vi "AAL NB Filter Specification.vi"(8 "timing jitter":enum32{"Interpolation", "Rounding"}(ring), 9 "stop band attenuation":dbl=2.0 format="%.2f", 11 "maximum decimation factor":i32) -> (1 "A stop [dB]":dbl=72.0 format="%.2f", 3 "decimation factor":i32)   [LabVIEW 2014, in "NI_AALPro.lvlib"]
uses:
  NI_AALPro.lvlib
panel:
  in  "force power of 2?":bool
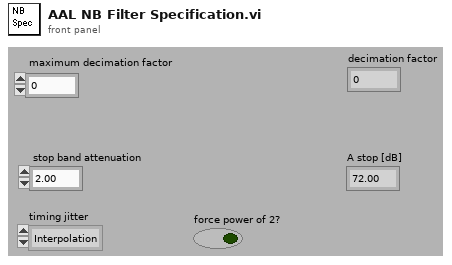
[diagram p1: front panel]
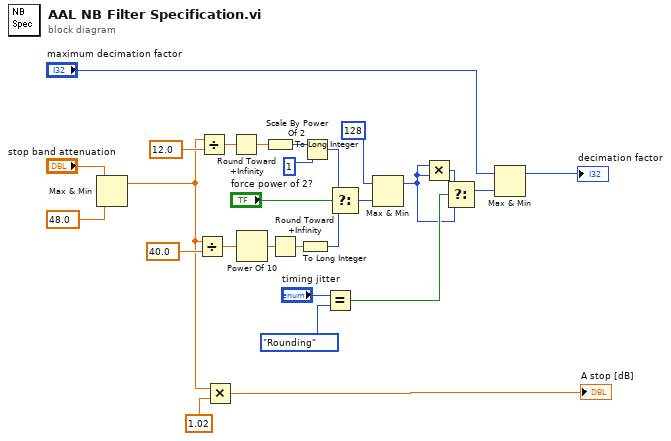
[diagram p0: block diagram]
diagram:
  n1 = Max & Min(x="stop band attenuation", y=48.0) -> (max(x,y)=w18:dbl)  [unwired: 1 out]
  n2 = Divide(x=w18, y=40.0) -> (x/y=w27:dbl)
  n3 = Divide(x=w18, y=12.0) -> (x/y=w20:dbl)
  n4 = Multiply(x=w18, y=1.02) -> (x*y=→"A stop [dB]":dbl)
  n5 = Round Toward +Infinity(x=w20) -> (ceil(x): smallest int >= x=w19:dbl)
  n6 = Power Of 10(x=w27) -> (10^x=w13:dbl)
  n7 = To Long Integer(number=w19) -> (32bit integer=w16:i32)
  n8 = Round Toward +Infinity(x=w13) -> (ceil(x): smallest int >= x=w14:dbl)
  n9 = To Long Integer(number=w14) -> (32bit integer=w12:i32)
  n10 = Scale By Power Of 2(n=w16, x=1) -> (x*2^n=w11:i32)
  n11 = Equal?(x="timing jitter", y=enum32{"Interpolation", "Rounding"}."Rounding") -> (x = y?=w6:bool)
  n12 = Select(t=w11, s="force power of 2?", f=w12) -> (s? t:f=w9:i32)
  n13 = Max & Min(x=128, y=w9) -> (max(x,y)=w1:i32)  [unwired: 1 out]
  n14 = Multiply(x=w1, y=w1) -> (x*y=w23:i32)
  n15 = Select(t=w23, s=w6, f=w1) -> (s? t:f=w4:i32)
  n16 = Max & Min(x="maximum decimation factor", y=w4) -> (max(x,y)=→"decimation factor":i32)  [unwired: 1 out]
